vi "Calc Roll.vi"(8 "y":dbl, 10 "Position":dbl) -> (2 "Roll":dbl)   [LabVIEW 2014]
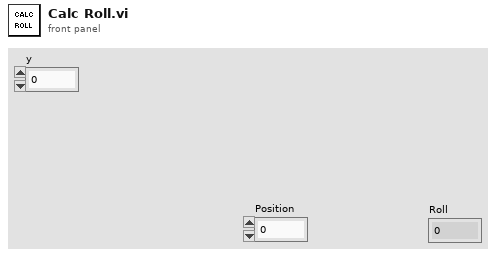
[diagram p1: front panel]
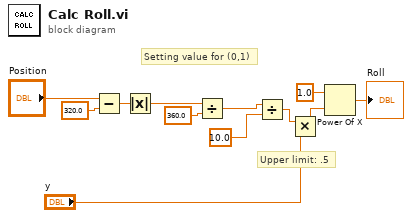
[diagram p0: block diagram]
diagram:
  # "Upper limit: .5"
  # "Setting value for (0,1)"
  n1 = Subtract(x="Position", y=320.0) -> (x-y=w10:dbl)
  n2 = Absolute Value(x=w10) -> (abs(x)=w9:dbl)
  n3 = Divide(x=w9, y=360.0) -> (x/y=w5:dbl)
  n4 = Divide(x=w5, y=10.0) -> (x/y=w3:dbl)
  n5 = Multiply(x=w3, y="y") -> (x*y=w2:dbl)
  n6 = Power Of X(1:w2, 2:1.0 ("y")) -> (0:→"Roll":dbl)
